vi "Test Server Stress.vi"() -> ()   [LabVIEW 2020]
uses:
  41ac7609-5d0e-48bc-9034-e5839c72e2f8.vi
  b4702106-43b1-43e1-a377-b71557efabfc.vi
  <vilib>/numeric/Random Number (Range) I64.vi
  source/Server/Server/Server.lvclass
  9482b7cb-b3ef-41c9-89c9-ae94feccced8.vi
  source/Value/Type Code.ctl
  source/Value/Value.lvlib
panel:
  in  "Instances of each type":i32=1 min=1 max=10000
  out "Array":T2(array[cluster])
  in  "Update":bool caption="Update values"
  in  "stop":bool
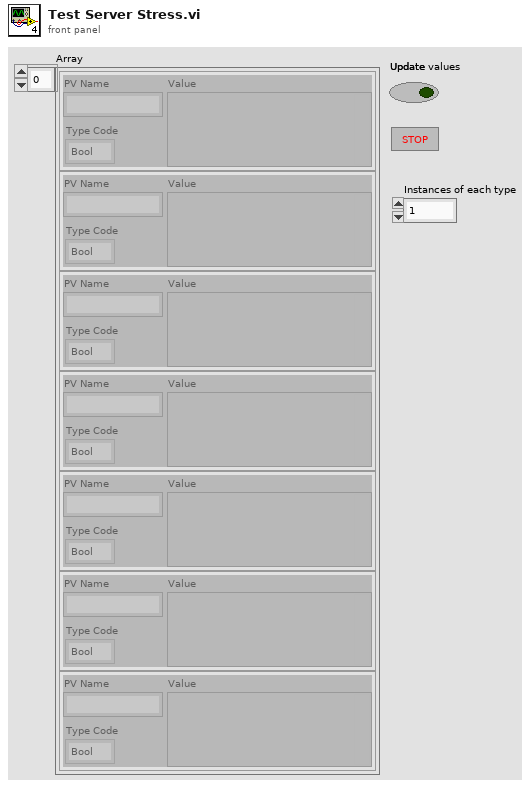
[diagram p1: front panel]
types:
  T1 = typedef "Value.lvlib/Type Code.ctl" = enum8{"Null", "Bool", "BoolA", "Int8", "Int8A", "Int16", "Int16A", "Int32", "Int32A", "Int64", "Int64A", "UInt8", "UInt8A", "UInt16", "UInt16A", "UInt32", "UInt32A", "UInt64", "UInt64A", "Float32", "Float32A", "Float64", "Float64A", "String", "StringA", "Struct", "StructA", "Union", "UnionA", "Any", "AnyA"}
  T2 = cluster{"PV Name":string, "Type Code":T1, "Value":variant}[]
  T3 = cluster{"output string":string, "Enum":T1, "value":variant}
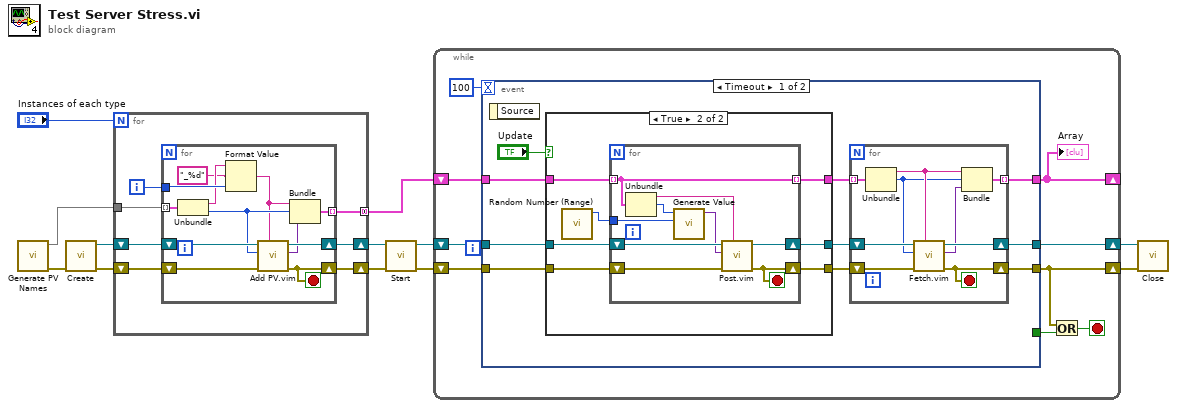
[diagram p0: block diagram]
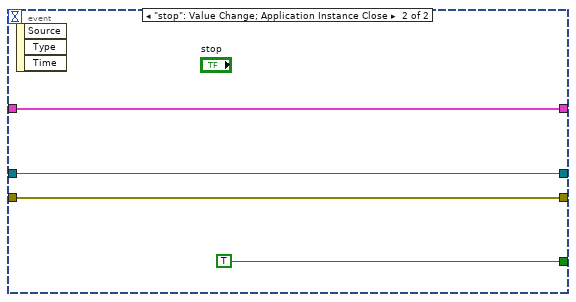
[diagram p3: hidden frame]
diagram:
  n1 = call "Generate PV Names.vi"() -> ("error out"=w6:errorcluster, "map"=w5:map{string, T1})  [unwired: 10 in]
  n2 = call "Create.vi"("error in (no error)"=w6) -> ("error out"=w8:errorcluster, "Server out"=w7:refnum<class "Server.lvclass">)  [unwired: 9 in]
  n3 = for {
    N: "Instances of each type" -> [_]
    tunnel: w5 -> [w15]
    tunnel: [w14] -> w2 mode=concatenating
    shift-right: [w19] -> w10
    shift-left: w8 -> [w17]
    shift-right: [w18] -> w9
    shift-left: w7 -> [w16]
    i -> [w13]
    n4 = for {
      tunnel: w15 -> [w31] mode=indexing
      shift-right: [w30] -> w18
      shift-left: w16 -> [w28]
      tunnel: [w26] -> w14 mode=indexing
      shift-right: [w24] -> w19
      shift-left: w17 -> [w29]
      tunnel: w13 -> [w23]
      stop <- w24 stop-if-true
      n5 = Unbundle(w31) -> (w22:string, "Enum"=w25:T1)
      n6 = Format Value(string ("")=w22, format string="_%d", value (0)=w23) -> (output string=w21:string)
      n7 = call "Add PV.vim"("PV name"=w21, "error in"=w29, "initial value"=w25, "Server in"=w28) -> ("error out"=w24:errorcluster, "value"=w27:variant, "Server out"=w30:refnum<class "Server.lvclass">)  [unwired: 5 in]
      n8 = Bundle("output string"=w21, "Enum"=w25, "value"=w27) -> (w26:T3)  [unwired: 1 in]
    }
  }
  n9 = call-dynamic "Start.vi"("error in (no error)"=w10, "Server in"=w9) -> ("error out"=w12:errorcluster, "Server out"=w11:refnum<class "Server.lvclass">)  [unwired: 8 in]
  n10 = while {
    shift-right: [w35] -> w4
    shift-left: w12 -> [w40]
    shift-right: [w38] -> w3
    shift-left: w11 -> [w39]
    shift-right: [w32] -> _
    shift-left: w2 -> [w33]
    stop <- w37 stop-if-true
    n11 = event shown="[0] Timeout" {
      selector: _ -> [_ _]
      dyn-events: _ -> [_ _]
      timeout: 100 -> [_ _]
      tunnel: [w41 w82] -> w35
      tunnel: w40 -> [w49 w82]
      tunnel: w39 -> [w50 w81]
      tunnel: [w42 w81] -> w38
      tunnel: [_ TRUE] -> w36
      tunnel: w33 -> [w47 w79]
      tunnel: [w43 w79] -> w32
      event Timeout {
        n12 = event-data() -> ()  [unwired: 1 in, 1 out]
        n13 = case shown="True" "Update" {
          tunnel: w50 -> [w62 w69]
          tunnel: [w62 w68] -> w45
          tunnel: w49 -> [w61 w67]
          tunnel: [w61 w66] -> w46
          tunnel: w47 -> [w60 w64]
          tunnel: [w60 w63] -> w44
          frame False {
          }
          frame True {
            n14 = call-poly <vilib>:"Random Number (Range).vi"() -> ("number"=w65:i64)  [unwired: 11 in]
            n15 = for {
              shift-right: [w74] -> w66
              shift-left: w67 -> [w76]
              tunnel: w64 -> [w70] mode=indexing
              shift-right: [w78] -> w68
              shift-left: w69 -> [w75]
              tunnel: w65 -> [w77]
              tunnel: [w70] -> w63 mode=indexing
              stop <- w74 stop-if-true
              n16 = Unbundle(w70) -> ("output string"=w73:string, "Enum"=w72:T1)  [unwired: 1 out]
              n17 = call "Generate Value.vi"("base value"=w77, "type code"=w72) -> ("value"=w71:variant)  [unwired: 9 in]
              n18 = call "Post.vim"("PV name"=w73, "error in"=w76, "value in"=w71, "Server in"=w75) -> ("error out"=w74:errorcluster, "Server out"=w78:refnum<class "Server.lvclass">)  [unwired: 5 in, 1 out]
            }
          }
        }
        n19 = for {
          shift-right: [w57] -> w42
          shift-left: w45 -> [w59]
          shift-right: [w56] -> w41
          shift-left: w46 -> [w58]
          tunnel: w44 -> [w55] mode=indexing
          tunnel: [w52] -> w43 mode=indexing
          stop <- w56 stop-if-true
          n20 = Unbundle(w55) -> ("output string"=w54:string, "Enum"=w51:T1)  [unwired: 1 out]
          n21 = call "Fetch.vim"("PV name"=w54, "error in"=w58, "default"=w51, "Server in"=w59) -> ("error out"=w56:errorcluster, "value"=w53:variant, "Server out"=w57:refnum<class "Server.lvclass">)  [unwired: 5 in]
          n22 = Bundle("output string"=w54, "Enum"=w51, "value"=w53) -> (w52:T3)  [unwired: 1 in]
        }
      }
      event "stop": Value Change; Application Instance Close {
        n23 = event-data() -> ()  [unwired: 1 in, 3 out]
      }
    }
    "Array" <- w32
    n24 = Or(x=w35, y=w36) -> (x .or. y?=w37:bool)
  }
  n25 = call-dynamic "Close.vi"("error in"=w4, "Server in"=w3) -> ()  [unwired: 9 in, 1 out]
